vi "Pre Launch Init.vi"(11 "Nested in":refnum<class "Soda Actor.lvclass">) -> (0 "error out":errorcluster, 3 "Nested out":refnum<class "Soda Actor.lvclass">)   [LabVIEW 2020, in "Soda Actor.lvlib" / "Soda Actor.lvclass"]
doc: "(<B>Filename</B>: Actor Framework.lvlib:Actor.lvclass:Pre Launch Init.vi)\n\nDefines behavior that occurs after the Launch Nested Actor method is invoked but before the actor's Actor Core method begins running.\n\nBy default, this method does nothing. A descendant class may override it to define behavior."
uses:
  Soda Actor.lvclass
  <vilib>/ActorFramework/Actor/Actor.lvclass
  Soda Actor Messages/init Msg/init Msg.lvclass
  C:/Program Files (x86)/National Instruments/LabVIEW 2020/vi.lib/ActorFramework/Actor/Actor.lvclass
  C:/Users/danie/Desktop/LabView/AF Proyect 2ndPartial/Proyecto-2do-parcial/AF 2Parcial/Soda Actor/Soda Actor.lvclass
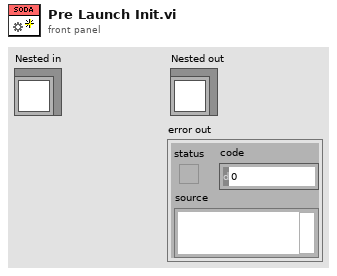
[diagram p1: front panel]
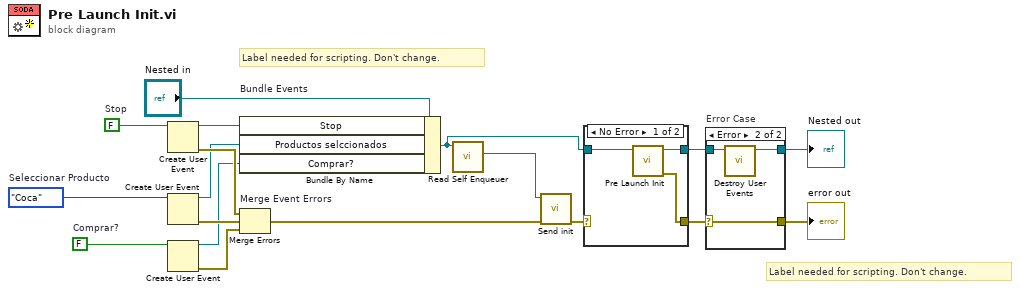
[diagram p0: block diagram]
diagram:
  w3 = FALSE  # Comprar?
  w6 = enum16{"Coca", "Fanta", "Manzanita", "Ciel"}."Coca"  # Seleccionar Producto
  w17 = FALSE  # Stop
  # "Label needed for scripting. Don't change."
  # "Label needed for scripting. Don't change."
  n1 = Create User Event(user event datatype=w17) -> (user event=w14:refnum<user-event>, error out=w16:errorcluster)  [unwired: 1 in]
  n2 = Create User Event(user event datatype=w6) -> (user event=w5:refnum<user-event>, error out=w4:errorcluster)  [unwired: 1 in]
  n3 = Create User Event(user event datatype=w3) -> (user event=w2:refnum<user-event>, error out=w1:errorcluster)  [unwired: 1 in]
  n4 = Bundle By Name "Bundle Events"(cluster="Nested in", "Stop"=w14, "Productos selccionados"=w5, "Comprar?"=w2) -> (w10:refnum<class "Soda Actor.lvclass">)
  n5 = Merge Errors "Merge Event Errors"(w16, w4, w1) -> (w8:errorcluster)
  n6 = call <vilib>:"Read Self Enqueuer.vi"("Actor"=w10) -> ("Self Enqueuer"=w9:refnum<class "Message Enqueuer.lvclass">)  [unwired: 10 in]
  n7 = call "Send init.vi"("error in (no error)"=w8, "Message Enqueuer"=w9) -> ("error out"=w7:errorcluster)  [unwired: 8 in, 1 out]
  n8 = case shown="No Error" w7 {
    selector: w7 -> [_ w23]
    tunnel: [w21 w22] -> w12
    tunnel: w10 -> [w20 w22]
    tunnel: [w19 w23] -> w11
    frame No Error {
      n9 = call-parent "Pre Launch Init.vi"("Actor in"=w20) -> ("error out"=w19:errorcluster, "Actor out"=w21:refnum<class "Soda Actor.lvclass">)  [unwired: 9 in]
    }
    frame Error {
    }
  }
  n10 = case "Error Case" shown="Error" w11 {
    selector: w11 -> [w24 w28]
    tunnel: w12 -> [w25 w27]
    tunnel: [w25 w26] -> w15
    tunnel: [w24 w28] -> w13
    frame No Error {
    }
    frame Error {
      n11 = call "Destroy User Events.vi"("UI Template in"=w27) -> ("UI Template out"=w26:refnum<class "Soda Actor.lvclass">)  [unwired: 10 in]
    }
  }
  "error out" <- w13
  "Nested out" <- w15
